vi "PressureSample.vi"(8 "error in (no error)":errorcluster, 11 "DAQREFS":T1) -> (0 "error out":errorcluster, 2 "Voltage":dbl format="%0.2f", 3 "DAQREFs":T1)   [LabVIEW 2021]
uses:
  Muscle Actuator LabV Analog/Controls/DAQ Refnums.ctl
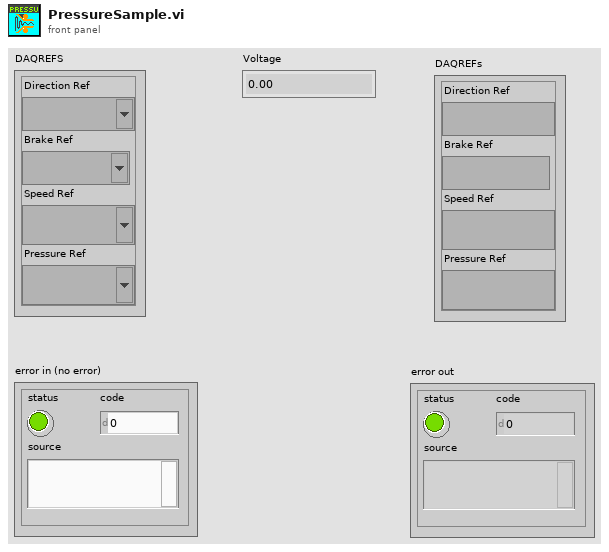
[diagram p1: front panel]
types:
  T1 = typedef "DAQ Refnums.ctl" = cluster{"Direction Ref":refnum<k21>, "Brake Ref":refnum<k21>, "Speed Ref":refnum<k21>, "Pressure Ref":refnum<k21>}
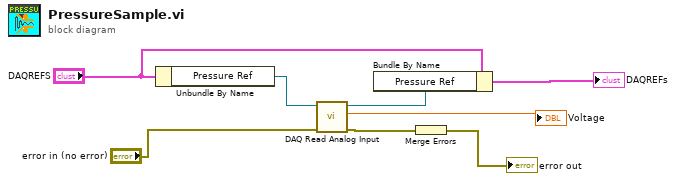
[diagram p0: block diagram]
diagram:
  n1 = Unbundle By Name("DAQREFS") -> ("Pressure Ref"=w3:refnum<k21>)
  n2 = call "DAQ Read Analog Input.vi"("error in"="error in (no error)", "task/channels in"=w3) -> ("error out"=w7:errorcluster, "Voltage"=→"Voltage":dbl, "task out"=w5:refnum<k21>)  [unwired: 7 in]
  n3 = Bundle By Name(cluster="DAQREFS", "Pressure Ref"=w5) -> (→"DAQREFs":T1)
  n4 = Merge Errors(w7) -> (→"error out":errorcluster)
